vi "首页.vi"() -> ()   [LabVIEW 2016]
uses:
  <vilib>/Utility/miscctls.llb/LVPointTypeDef.ctl
  <vilib>/Utility/sysdir.llb/System Directory Type.ctl
  <vilib>/addons/database/_DB Variant To Data/Database Variant To Data.xnode
panel:
  out "显示":T1
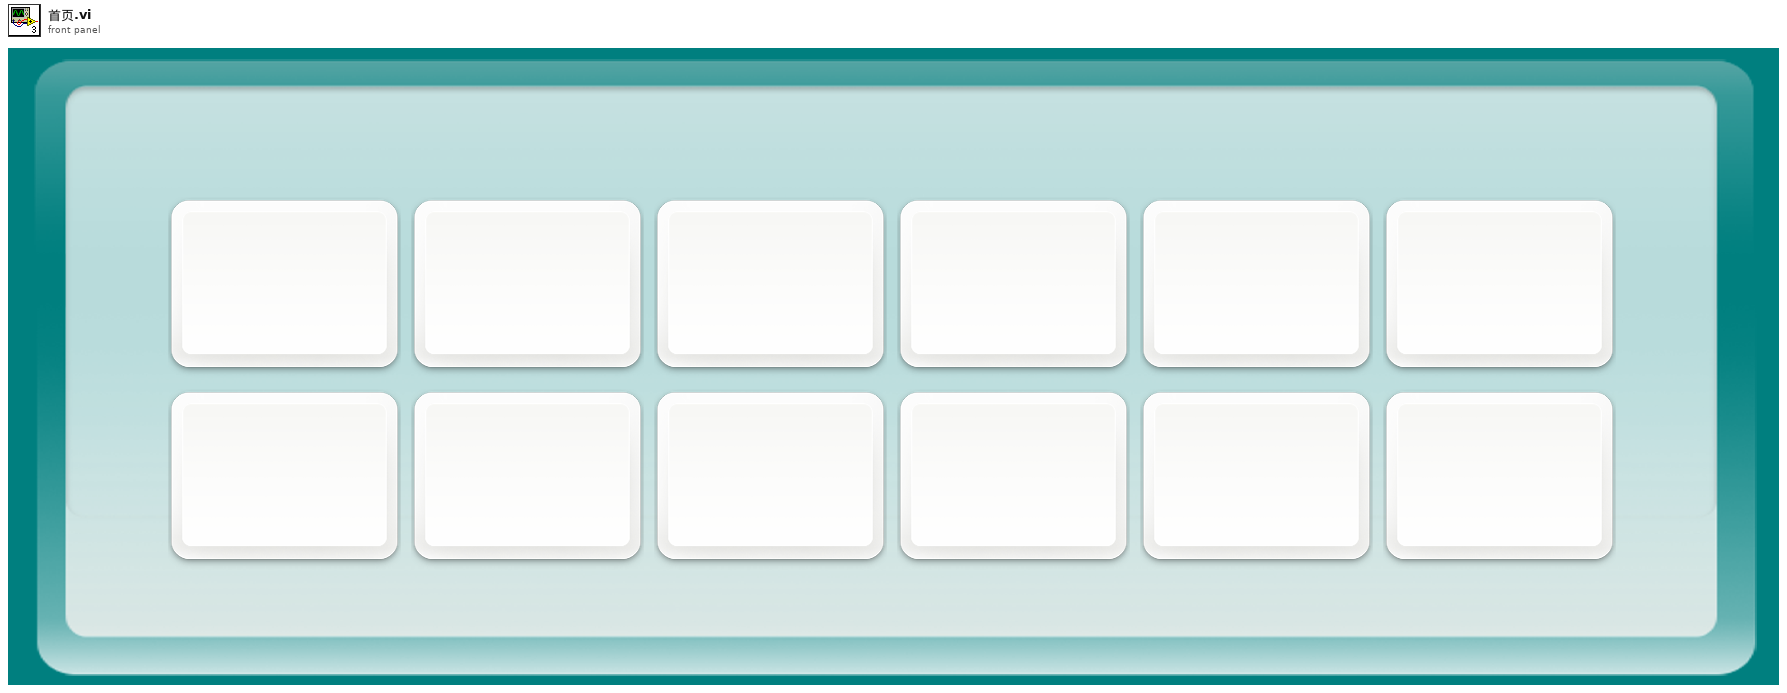
[diagram p1: front panel]
types:
  T1 = typedef "多数值显示.ctl" = cluster{"显示":T2, "显示 2":T2, "显示 3":T2, "显示 4":T2, "显示 5":T2, "显示 6":T2, "显示 12":T2, "显示 11":T2, "显示 10":T2, "显示 9":T2, "显示 8":T2, "显示 7":T2}
  T2 = typedef "数值显示.ctl" = cluster{"中文项目名称":string, "英文项目名称":string, "浓度":string, "单位":string}
  T3 = typedef "LVPointTypeDef.ctl" = cluster{"Horizontal":i16, "Vertical":i16}
  T4 = cluster{"显示参数中文名":string, "显示参数英文名":string, "显示浓度":string, "显示单位":string}[]
  T5 = cluster{"显示参数中文名":string, "显示参数英文名":string, "显示浓度":string, "显示单位":string}
  T6 = typedef "System Directory Type.ctl" = i32
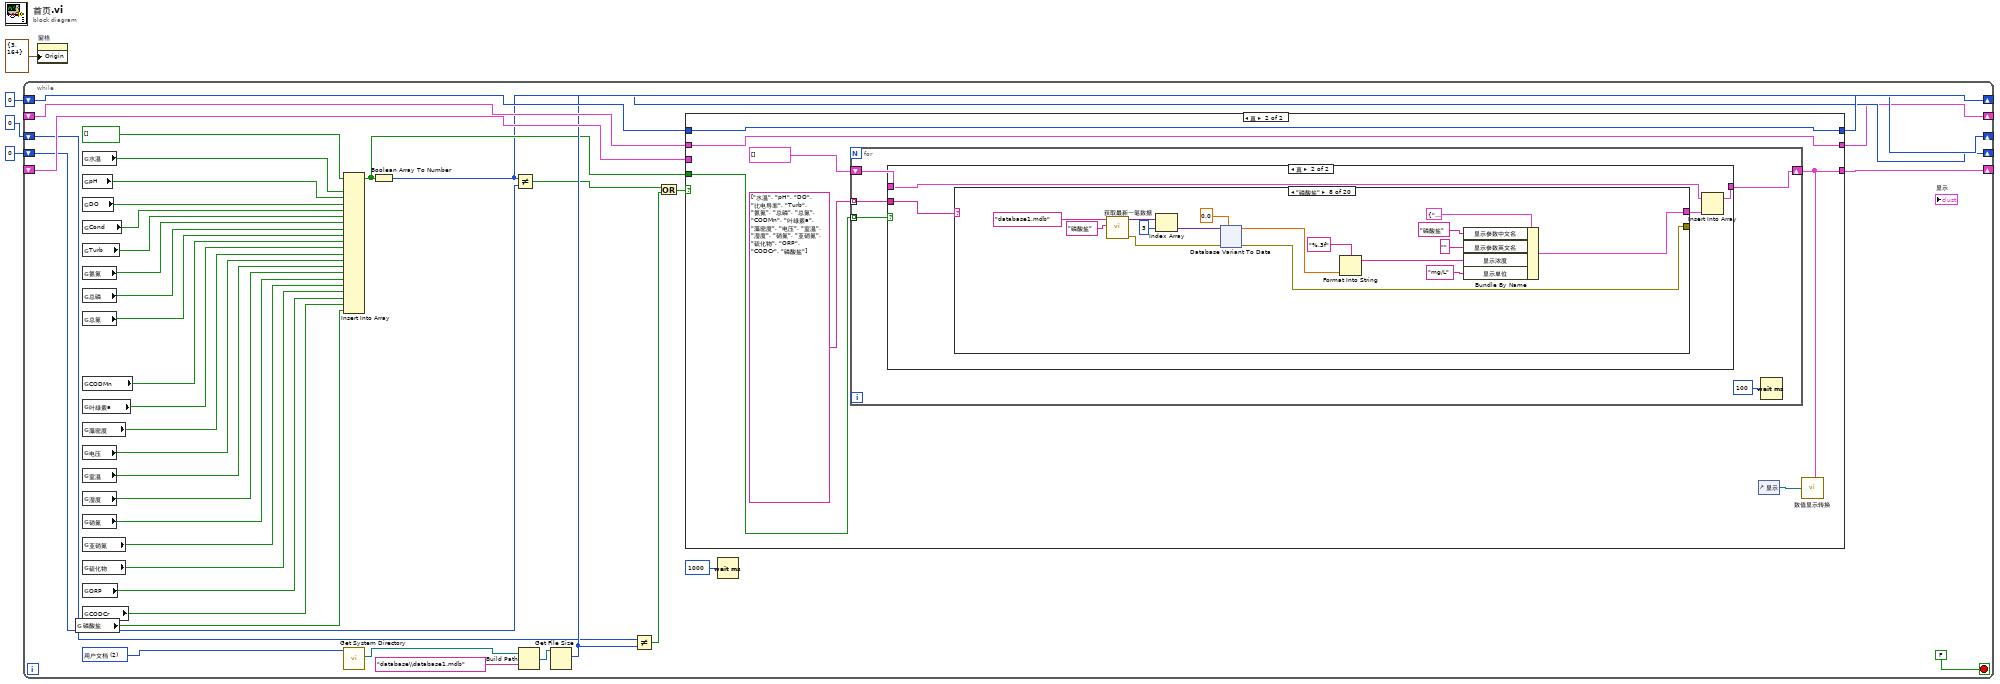
[diagram p0: block diagram]
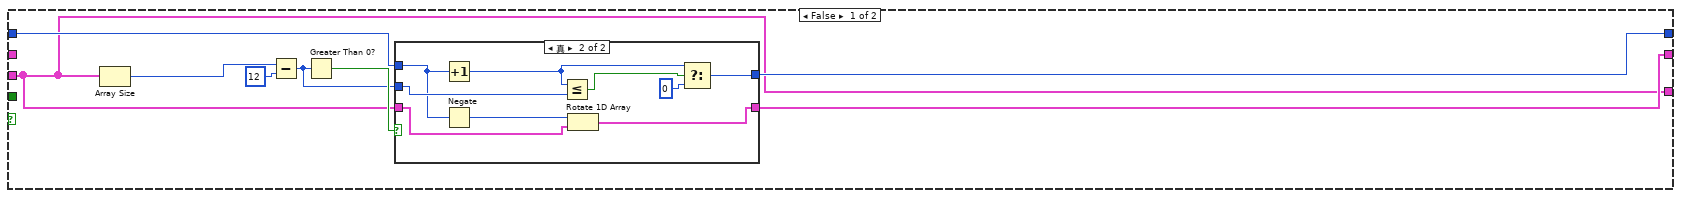
[diagram p2: hidden frame]
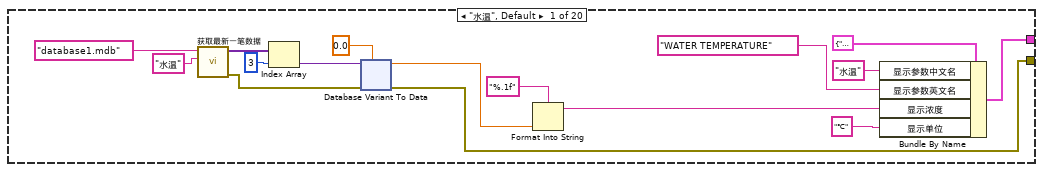
[diagram p5: hidden frame]
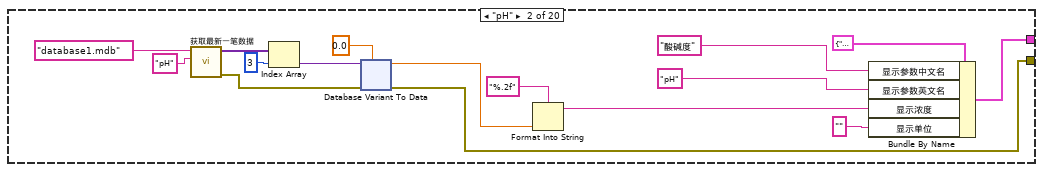
[diagram p6: hidden frame]
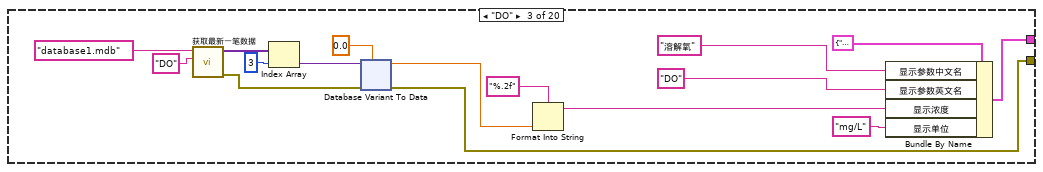
[diagram p7: hidden frame]
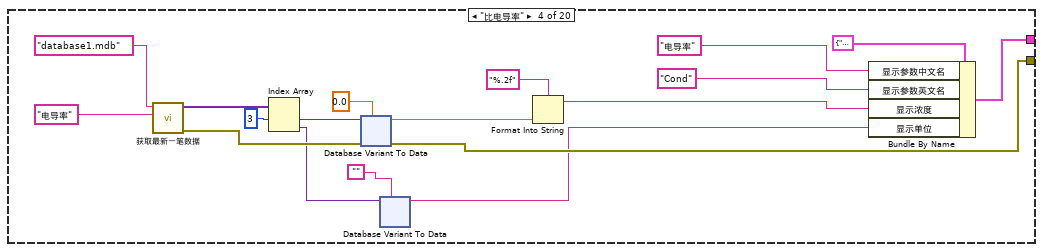
[diagram p8: hidden frame]
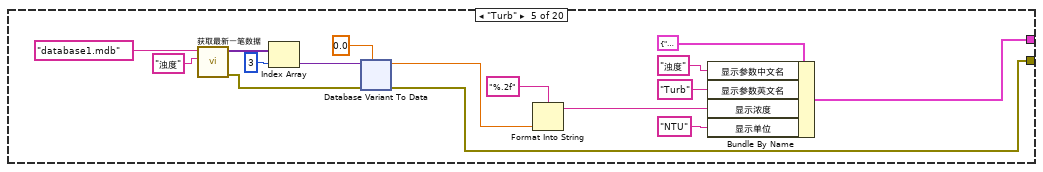
[diagram p9: hidden frame]
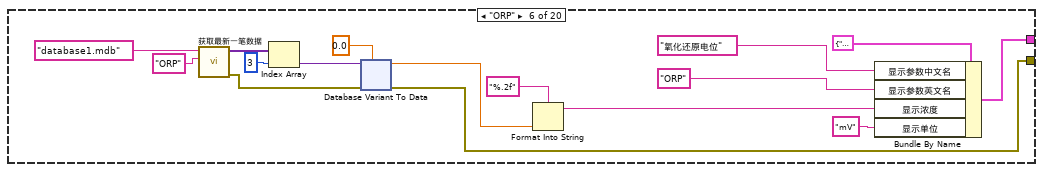
[diagram p10: hidden frame]
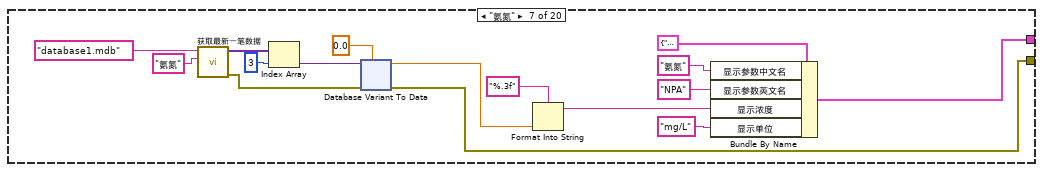
[diagram p11: hidden frame]
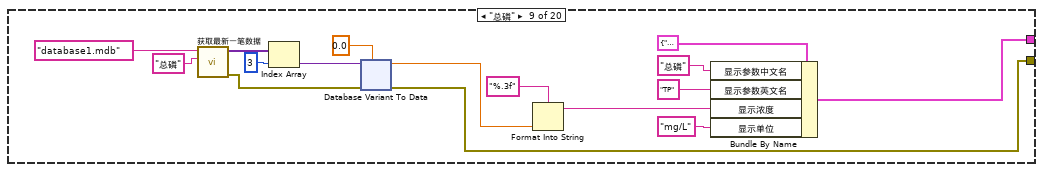
[diagram p12: hidden frame]
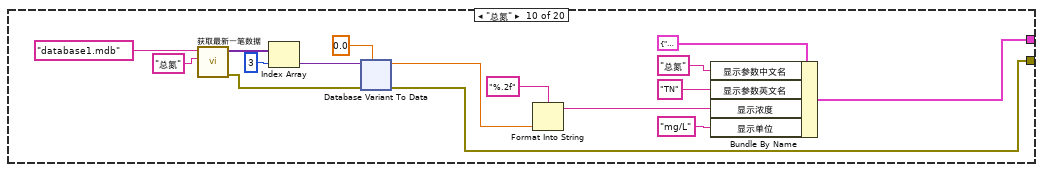
[diagram p13: hidden frame]
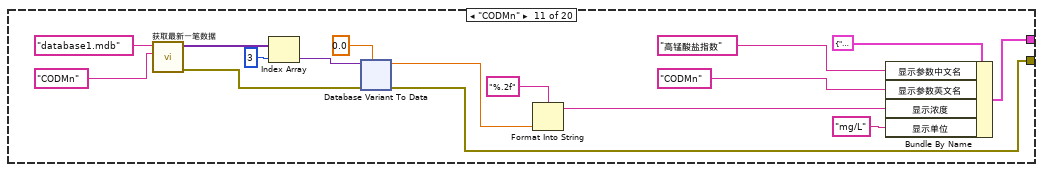
[diagram p14: hidden frame]
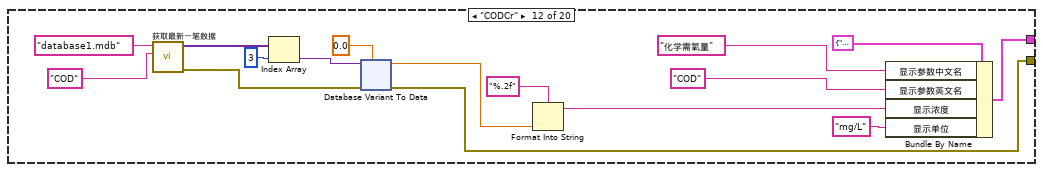
[diagram p15: hidden frame]
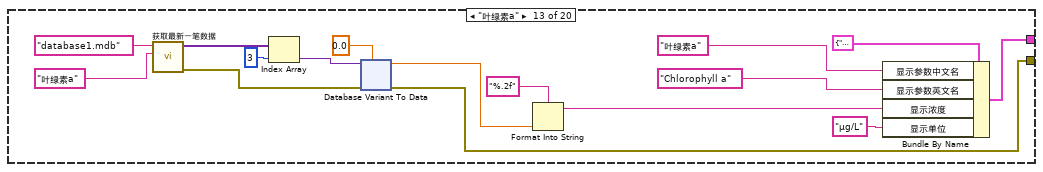
[diagram p16: hidden frame]
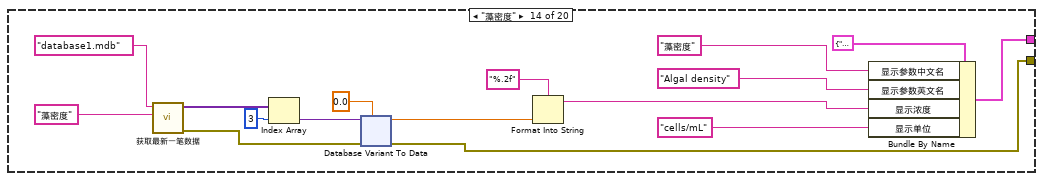
[diagram p17: hidden frame]
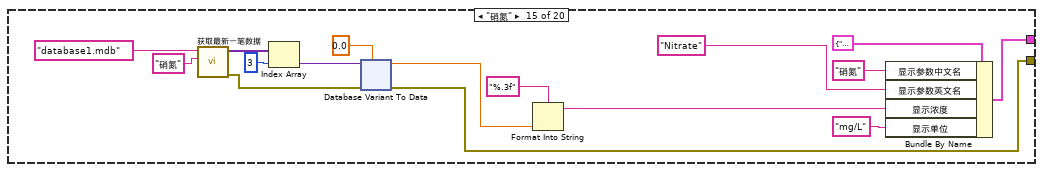
[diagram p18: hidden frame]
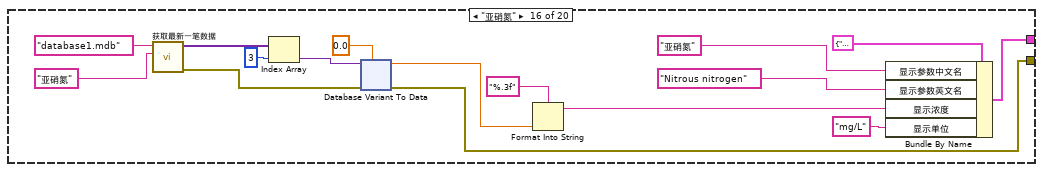
[diagram p19: hidden frame]
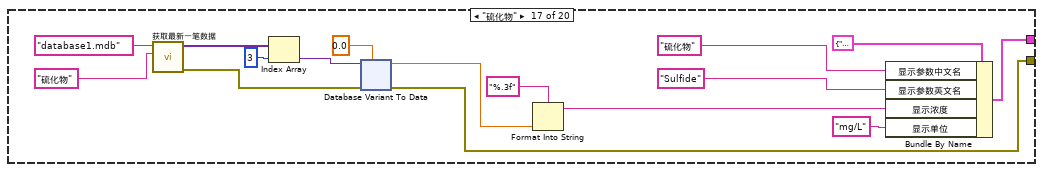
[diagram p20: hidden frame]
diagram:
  n1 = while {
    shift-right: [w43] -> _
    shift-left: _ -> [w42]
    shift-right: [w41] -> _
    shift-left: 0 -> [w44]
    shift-right: [w6] -> _
    shift-left: _ -> [w40]
    shift-right: [w35] -> _
    shift-left: i64 0 ("size (in bytes)") -> [w34]
    shift-right: [w13] -> _
    shift-left: u32 0 -> [w12]
    stop <- FALSE stop-if-true
    w39 = T6 2 items=["用户目录"=0, "用户桌面"=1, "用户文档"=2, "用户应用程序数据"=3, "用户设置"=4, "用户临时目录"=5, "公共文档"=6, "公共应用程序数据"=7, "公共设置"=8, "公共缓存"=13, "系统核心库"=9, "系统安装库"=10, "应用程序文件"=11, "启动盘根目录"=12] ("system directory type")
    n2 = global read "首页设置全局变量.vi" "磷酸盐"() -> (w5:bool)
    n3 = global read "首页设置全局变量.vi" "水温"() -> (w27:bool)
    n4 = global read "首页设置全局变量.vi" "pH"() -> (w26:bool)
    n5 = global read "首页设置全局变量.vi" "DO"() -> (w25:bool)
    n6 = global read "首页设置全局变量.vi" "Cond"() -> (w24:bool)
    n7 = global read "首页设置全局变量.vi" "Turb"() -> (w23:bool)
    n8 = global read "首页设置全局变量.vi" "氨氮"() -> (w22:bool)
    n9 = global read "首页设置全局变量.vi" "总磷"() -> (w21:bool)
    n10 = global read "首页设置全局变量.vi" "总氮"() -> (w20:bool)
    n11 = global read "首页设置全局变量.vi" "CODMn"() -> (w19:bool)
    n12 = global read "首页设置全局变量.vi" "叶绿素a"() -> (w18:bool)
    n13 = global read "首页设置全局变量.vi" "藻密度"() -> (w17:bool)
    n14 = global read "首页设置全局变量.vi" "电压"() -> (w16:bool)
    n15 = global read "首页设置全局变量.vi" "室温"() -> (w15:bool)
    n16 = global read "首页设置全局变量.vi" "湿度"() -> (w29:bool)
    n17 = global read "首页设置全局变量.vi" "硝氮"() -> (w30:bool)
    n18 = global read "首页设置全局变量.vi" "亚硝氮"() -> (w31:bool)
    n19 = global read "首页设置全局变量.vi" "硫化物"() -> (w32:bool)
    n20 = global read "首页设置全局变量.vi" "ORP"() -> (w33:bool)
    n21 = global read "首页设置全局变量.vi" "CODCr"() -> (w7:bool)
    n22 = Insert Into Array(array=bool[] [], new element #1=w27, new element #2=w26, new element #3=w25, new element #4=w24, new element #5=w23, new element #6=w22, new element #7=w21, new element #8=w20, new element #9=w19, new element #10=w18, new element #11=w17, new element #12=w16, new element #13=w15, new element #14=w29, new element #15=w30, new element #16=w31, new element #17=w32, new element #18=w33, new element #19=w7, new element #20=w5) -> (w14:bool[])  [unwired: 1 in]
    n23 = call <vilib>:"Get System Directory.vi"("system directory type"=w39) -> ("system directory"=w38:path)  [unwired: 10 in]
    n24 = Boolean Array To Number(Boolean array=w14) -> (number=w13:u32)
    n25 = Not Equal?(x=w13, y=w12) -> (x != y?=w11:bool)
    n26 = Build Path(base path=w38, name or relative path="database\\database1.mdb" ("名称或相对路径")) -> (appended path=w36:path)
    n27 = Get File Size(file=w36) -> (size (in bytes)=w35:i64)  [unwired: 1 in, 2 out]
    n28 = Not Equal?(x=w34, y=w35) -> (x != y?=w10:bool)
    n29 = Or(x=w11, y=w10) -> (x .or. y?=w9:bool)
    n30 = case shown="真" w9 {
      tunnel: w44 -> [w53 w68]
      tunnel: [w46 w64] -> w43
      tunnel: w42 -> [w46 _]
      tunnel: [w52 w68] -> w41
      tunnel: [w47 w67] -> w6
      tunnel: w40 -> [_ w67]
      tunnel: w14 -> [_ w66]
      frame False {
        n31 = Array Size(array=w46) -> (size(s)=w51:i32)
        n32 = Subtract(x=w51, y=12) -> (x-y=w48:i32)
        n33 = Greater Than 0?(x=w48) -> (x > 0?=w49:bool)
        n34 = case shown="真" w49 {
          tunnel: w46 -> [w54 w63]
          tunnel: w53 -> [_ w56]
          tunnel: [w54 w62] -> w47
          tunnel: [_ w57] -> w52
          tunnel: w48 -> [_ w60]
          frame False {
          }
          frame True {
            n35 = Increment(x=w56) -> (x+1=w61:i32)
            n36 = Negate(x=w56) -> (-x=w55:i32)
            n37 = Less Or Equal?(x=w61, y=w60) -> (x <= y?=w59:bool)
            n38 = Rotate 1D Array(1:w63, 2:w55) -> (0:w62:T4)
            n39 = Select(t=w61, s=w59, f=0) -> (s? t:f=w57:i32)
          }
        }
      }
      frame True {
        n40 = for {
          tunnel: w66 -> [w75] mode=indexing
          tunnel: string[] ["水温", "pH", "DO", "比电导率", "Turb", "氨氮", "总磷", "总氮", "CODMn", "叶绿素a", "藻密度", "电压", "室温", "湿度", "硝氮", "亚硝氮", "硫化物", "ORP", "CODCr", "磷酸盐"] -> [w74] mode=indexing
          shift-right: [w72] -> w64
          shift-left: T4 [] -> [w73]
          n41 = case shown="真" w75 {
            tunnel: w74 -> [_ w80]
            tunnel: w73 -> [w76 w79]
            tunnel: [w76 w78] -> w72
            frame False {
            }
            frame True {
              n42 = case shown="\"磷酸盐\"" w80 {
                tunnel: [w90 w140 w188 w239 w318 w366 w414 w462 w510 w558 w606 w654 w702 w750 w798 w846 w894 w934 w942 w950] -> w77
                tunnel: [w89 w137 w185 w235 w314 w362 w403 w451 w499 w547 w595 w643 w698 w739 w787 w835 w883 _ _ _] -> _
                frame "水温", Default {
                  n43 = call "获取最新一笔数据.vi"("table"="水温", "database"="database1.mdb" ("名称或相对路径")) -> ("error out"=w81:errorcluster, "子数组"=w86:variant[])  [unwired: 8 in]
                  n44 = Index Array(array=w86, index=3 ("索引")) -> (element=w84:variant)
                  n45 = xnode "Database Variant To Data"("database variant"=w84, "error in (no error)"=w81, "type"=0.0) -> ("data"=w88:dbl, "error out"=w89:errorcluster)
                  n46 = Format Into String(format string="%.1f" ("格式字符串"), w88) -> (resulting string=w91:string)  [unwired: 2 in, 1 out]
                  n47 = Bundle By Name(cluster=T5 {"显示参数中文名"="", "显示参数英文名"="", "显示浓度"="", "显示单位"=""} ("元素"), "显示参数中文名"="水温", "显示参数英文名"="WATER TEMPERATURE", "显示浓度"=w91, "显示单位"="℃") -> (w90:T5)
                }
                frame "pH" {
                  n48 = call "获取最新一笔数据.vi"("table"="pH", "database"="database1.mdb" ("名称或相对路径")) -> ("error out"=w129:errorcluster, "子数组"=w134:variant[])  [unwired: 8 in]
                  n49 = Index Array(array=w134, index=3 ("索引")) -> (element=w132:variant)
                  n50 = xnode "Database Variant To Data"("database variant"=w132, "error in (no error)"=w129, "type"=0.0) -> ("data"=w136:dbl, "error out"=w137:errorcluster)
                  n51 = Format Into String(format string="%.2f" ("格式字符串"), w136) -> (resulting string=w138:string)  [unwired: 2 in, 1 out]
                  n52 = Bundle By Name(cluster=T5 {"显示参数中文名"="", "显示参数英文名"="", "显示浓度"="", "显示单位"=""} ("元素"), "显示参数中文名"="酸碱度", "显示参数英文名"="pH", "显示浓度"=w138, "显示单位"="") -> (w140:T5)
                }
                frame "DO" {
                  n53 = call "获取最新一笔数据.vi"("table"="DO", "database"="database1.mdb" ("名称或相对路径")) -> ("error out"=w177:errorcluster, "子数组"=w182:variant[])  [unwired: 8 in]
                  n54 = Index Array(array=w182, index=3 ("索引")) -> (element=w180:variant)
                  n55 = xnode "Database Variant To Data"("database variant"=w180, "error in (no error)"=w177, "type"=0.0) -> ("data"=w184:dbl, "error out"=w185:errorcluster)
                  n56 = Format Into String(format string="%.2f" ("格式字符串"), w184) -> (resulting string=w186:string)  [unwired: 2 in, 1 out]
                  n57 = Bundle By Name(cluster=T5 {"显示参数中文名"="", "显示参数英文名"="", "显示浓度"="", "显示单位"=""} ("元素"), "显示参数中文名"="溶解氧", "显示参数英文名"="DO", "显示浓度"=w186, "显示单位"="mg/L") -> (w188:T5)
                }
                frame "比电导率" {
                  n58 = call "获取最新一笔数据.vi"("table"="电导率", "database"="database1.mdb" ("名称或相对路径")) -> ("error out"=w228:errorcluster, "子数组"=w233:variant[])  [unwired: 8 in]
                  n59 = Index Array(array=w233, index #1=3 ("索引")) -> (element #1=w231:variant, element #2=w227:variant)  [unwired: 1 in]
                  n60 = xnode "Database Variant To Data"("database variant"=w231, "error in (no error)"=w228, "type"=0.0) -> ("data"=w236:dbl, "error out"=w235:errorcluster)
                  n61 = xnode "Database Variant To Data"("database variant"=w227, "type"="") -> ("data"=w225:string)  [unwired: 1 in, 1 out]
                  n62 = Format Into String(format string="%.2f" ("格式字符串"), w236) -> (resulting string=w237:string)  [unwired: 2 in, 1 out]
                  n63 = Bundle By Name(cluster=T5 {"显示参数中文名"="", "显示参数英文名"="", "显示浓度"="", "显示单位"=""} ("元素"), "显示参数中文名"="电导率", "显示参数英文名"="Cond", "显示浓度"=w237, "显示单位"=w225) -> (w239:T5)
                }
                frame "Turb" {
                  n64 = call "获取最新一笔数据.vi"("table"="浊度", "database"="database1.mdb" ("名称或相对路径")) -> ("error out"=w307:errorcluster, "子数组"=w312:variant[])  [unwired: 8 in]
                  n65 = Index Array(array=w312, index=3 ("索引")) -> (element=w310:variant)
                  n66 = xnode "Database Variant To Data"("database variant"=w310, "error in (no error)"=w307, "type"=0.0) -> ("data"=w315:dbl, "error out"=w314:errorcluster)
                  n67 = Format Into String(format string="%.2f" ("格式字符串"), w315) -> (resulting string=w316:string)  [unwired: 2 in, 1 out]
                  n68 = Bundle By Name(cluster=T5 {"显示参数中文名"="", "显示参数英文名"="", "显示浓度"="", "显示单位"=""} ("元素"), "显示参数中文名"="浊度", "显示参数英文名"="Turb", "显示浓度"=w316, "显示单位"="NTU") -> (w318:T5)
                }
                frame "ORP" {
                  n69 = call "获取最新一笔数据.vi"("table"="ORP", "database"="database1.mdb" ("名称或相对路径")) -> ("error out"=w355:errorcluster, "子数组"=w360:variant[])  [unwired: 8 in]
                  n70 = Index Array(array=w360, index=3 ("索引")) -> (element=w358:variant)
                  n71 = xnode "Database Variant To Data"("database variant"=w358, "error in (no error)"=w355, "type"=0.0) -> ("data"=w363:dbl, "error out"=w362:errorcluster)
                  n72 = Format Into String(format string="%.2f" ("格式字符串"), w363) -> (resulting string=w364:string)  [unwired: 2 in, 1 out]
                  n73 = Bundle By Name(cluster=T5 {"显示参数中文名"="", "显示参数英文名"="", "显示浓度"="", "显示单位"=""} ("元素"), "显示参数中文名"="氧化还原电位", "显示参数英文名"="ORP", "显示浓度"=w364, "显示单位"="mV") -> (w366:T5)
                }
                frame "氨氮" {
                  n74 = call "获取最新一笔数据.vi"("table"="氨氮", "database"="database1.mdb" ("名称或相对路径")) -> ("error out"=w404:errorcluster, "子数组"=w410:variant[])  [unwired: 8 in]
                  n75 = Index Array(array=w410, index=3 ("索引")) -> (element=w408:variant)
                  n76 = xnode "Database Variant To Data"("database variant"=w408, "error in (no error)"=w404, "type"=0.0) -> ("data"=w405:dbl, "error out"=w403:errorcluster)
                  n77 = Format Into String(format string="%.3f" ("格式字符串"), w405) -> (resulting string=w412:string)  [unwired: 2 in, 1 out]
                  n78 = Bundle By Name(cluster=T5 {"显示参数中文名"="", "显示参数英文名"="", "显示浓度"="", "显示单位"=""} ("元素"), "显示参数中文名"="氨氮", "显示参数英文名"="NPA", "显示浓度"=w412, "显示单位"="mg/L") -> (w414:T5)
                }
                frame "磷酸盐" {
                  n79 = call "获取最新一笔数据.vi"("table"="磷酸盐", "database"="database1.mdb" ("名称或相对路径")) -> ("error out"=w452:errorcluster, "子数组"=w458:variant[])  [unwired: 8 in]
                  n80 = Index Array(array=w458, index=3 ("索引")) -> (element=w456:variant)
                  n81 = xnode "Database Variant To Data"("database variant"=w456, "error in (no error)"=w452, "type"=0.0) -> ("data"=w453:dbl, "error out"=w451:errorcluster)
                  n82 = Format Into String(format string="%.3f" ("格式字符串"), w453) -> (resulting string=w460:string)  [unwired: 2 in, 1 out]
                  n83 = Bundle By Name(cluster=T5 {"显示参数中文名"="", "显示参数英文名"="", "显示浓度"="", "显示单位"=""} ("元素"), "显示参数中文名"="磷酸盐", "显示参数英文名"="", "显示浓度"=w460, "显示单位"="mg/L") -> (w462:T5)
                }
                frame "总磷" {
                  n84 = call "获取最新一笔数据.vi"("table"="总磷", "database"="database1.mdb" ("名称或相对路径")) -> ("error out"=w500:errorcluster, "子数组"=w506:variant[])  [unwired: 8 in]
                  n85 = Index Array(array=w506, index=3 ("索引")) -> (element=w504:variant)
                  n86 = xnode "Database Variant To Data"("database variant"=w504, "error in (no error)"=w500, "type"=0.0) -> ("data"=w501:dbl, "error out"=w499:errorcluster)
                  n87 = Format Into String(format string="%.3f" ("格式字符串"), w501) -> (resulting string=w508:string)  [unwired: 2 in, 1 out]
                  n88 = Bundle By Name(cluster=T5 {"显示参数中文名"="", "显示参数英文名"="", "显示浓度"="", "显示单位"=""} ("元素"), "显示参数中文名"="总磷", "显示参数英文名"="TP", "显示浓度"=w508, "显示单位"="mg/L") -> (w510:T5)
                }
                frame "总氮" {
                  n89 = call "获取最新一笔数据.vi"("table"="总氮", "database"="database1.mdb" ("名称或相对路径")) -> ("error out"=w548:errorcluster, "子数组"=w554:variant[])  [unwired: 8 in]
                  n90 = Index Array(array=w554, index=3 ("索引")) -> (element=w552:variant)
                  n91 = xnode "Database Variant To Data"("database variant"=w552, "error in (no error)"=w548, "type"=0.0) -> ("data"=w549:dbl, "error out"=w547:errorcluster)
                  n92 = Format Into String(format string="%.2f" ("格式字符串"), w549) -> (resulting string=w556:string)  [unwired: 2 in, 1 out]
                  n93 = Bundle By Name(cluster=T5 {"显示参数中文名"="", "显示参数英文名"="", "显示浓度"="", "显示单位"=""} ("元素"), "显示参数中文名"="总氮", "显示参数英文名"="TN", "显示浓度"=w556, "显示单位"="mg/L") -> (w558:T5)
                }
                frame "CODMn" {
                  n94 = call "获取最新一笔数据.vi"("table"="CODMn", "database"="database1.mdb" ("名称或相对路径")) -> ("error out"=w596:errorcluster, "子数组"=w602:variant[])  [unwired: 8 in]
                  n95 = Index Array(array=w602, index=3 ("索引")) -> (element=w600:variant)
                  n96 = xnode "Database Variant To Data"("database variant"=w600, "error in (no error)"=w596, "type"=0.0) -> ("data"=w597:dbl, "error out"=w595:errorcluster)
                  n97 = Format Into String(format string="%.2f" ("格式字符串"), w597) -> (resulting string=w604:string)  [unwired: 2 in, 1 out]
                  n98 = Bundle By Name(cluster=T5 {"显示参数中文名"="", "显示参数英文名"="", "显示浓度"="", "显示单位"=""} ("元素"), "显示参数中文名"="高锰酸盐指数", "显示参数英文名"="CODMn", "显示浓度"=w604, "显示单位"="mg/L") -> (w606:T5)
                }
                frame "CODCr" {
                  n99 = call "获取最新一笔数据.vi"("table"="COD", "database"="database1.mdb" ("名称或相对路径")) -> ("error out"=w644:errorcluster, "子数组"=w650:variant[])  [unwired: 8 in]
                  n100 = Index Array(array=w650, index=3 ("索引")) -> (element=w648:variant)
                  n101 = xnode "Database Variant To Data"("database variant"=w648, "error in (no error)"=w644, "type"=0.0) -> ("data"=w645:dbl, "error out"=w643:errorcluster)
                  n102 = Format Into String(format string="%.2f" ("格式字符串"), w645) -> (resulting string=w652:string)  [unwired: 2 in, 1 out]
                  n103 = Bundle By Name(cluster=T5 {"显示参数中文名"="", "显示参数英文名"="", "显示浓度"="", "显示单位"=""} ("元素"), "显示参数中文名"="化学需氧量", "显示参数英文名"="COD", "显示浓度"=w652, "显示单位"="mg/L") -> (w654:T5)
                }
                frame "叶绿素a" {
                  n104 = call "获取最新一笔数据.vi"("table"="叶绿素a", "database"="database1.mdb" ("名称或相对路径")) -> ("error out"=w691:errorcluster, "子数组"=w696:variant[])  [unwired: 8 in]
                  n105 = Index Array(array=w696, index=3 ("索引")) -> (element=w694:variant)
                  n106 = xnode "Database Variant To Data"("database variant"=w694, "error in (no error)"=w691, "type"=0.0) -> ("data"=w699:dbl, "error out"=w698:errorcluster)
                  n107 = Format Into String(format string="%.2f" ("格式字符串"), w699) -> (resulting string=w700:string)  [unwired: 2 in, 1 out]
                  n108 = Bundle By Name(cluster=T5 {"显示参数中文名"="", "显示参数英文名"="", "显示浓度"="", "显示单位"=""} ("元素"), "显示参数中文名"="叶绿素a", "显示参数英文名"="Chlorophyll a", "显示浓度"=w700, "显示单位"="μg/L") -> (w702:T5)
                }
                frame "藻密度" {
                  n109 = call "获取最新一笔数据.vi"("table"="藻密度", "database"="database1.mdb" ("名称或相对路径")) -> ("error out"=w740:errorcluster, "子数组"=w746:variant[])  [unwired: 8 in]
                  n110 = Index Array(array=w746, index=3 ("索引")) -> (element=w744:variant)
                  n111 = xnode "Database Variant To Data"("database variant"=w744, "error in (no error)"=w740, "type"=0.0) -> ("data"=w741:dbl, "error out"=w739:errorcluster)
                  n112 = Format Into String(format string="%.2f" ("格式字符串"), w741) -> (resulting string=w748:string)  [unwired: 2 in, 1 out]
                  n113 = Bundle By Name(cluster=T5 {"显示参数中文名"="", "显示参数英文名"="", "显示浓度"="", "显示单位"=""} ("元素"), "显示参数中文名"="藻密度", "显示参数英文名"="Algal density", "显示浓度"=w748, "显示单位"="cells/mL") -> (w750:T5)
                }
                frame "硝氮" {
                  n114 = call "获取最新一笔数据.vi"("table"="硝氮", "database"="database1.mdb" ("名称或相对路径")) -> ("error out"=w788:errorcluster, "子数组"=w794:variant[])  [unwired: 8 in]
                  n115 = Index Array(array=w794, index=3 ("索引")) -> (element=w792:variant)
                  n116 = xnode "Database Variant To Data"("database variant"=w792, "error in (no error)"=w788, "type"=0.0) -> ("data"=w789:dbl, "error out"=w787:errorcluster)
                  n117 = Format Into String(format string="%.3f" ("格式字符串"), w789) -> (resulting string=w796:string)  [unwired: 2 in, 1 out]
                  n118 = Bundle By Name(cluster=T5 {"显示参数中文名"="", "显示参数英文名"="", "显示浓度"="", "显示单位"=""} ("元素"), "显示参数中文名"="硝氮", "显示参数英文名"="Nitrate", "显示浓度"=w796, "显示单位"="mg/L") -> (w798:T5)
                }
                frame "亚硝氮" {
                  n119 = call "获取最新一笔数据.vi"("table"="亚硝氮", "database"="database1.mdb" ("名称或相对路径")) -> ("error out"=w836:errorcluster, "子数组"=w842:variant[])  [unwired: 8 in]
                  n120 = Index Array(array=w842, index=3 ("索引")) -> (element=w840:variant)
                  n121 = xnode "Database Variant To Data"("database variant"=w840, "error in (no error)"=w836, "type"=0.0) -> ("data"=w837:dbl, "error out"=w835:errorcluster)
                  n122 = Format Into String(format string="%.3f" ("格式字符串"), w837) -> (resulting string=w844:string)  [unwired: 2 in, 1 out]
                  n123 = Bundle By Name(cluster=T5 {"显示参数中文名"="", "显示参数英文名"="", "显示浓度"="", "显示单位"=""} ("元素"), "显示参数中文名"="亚硝氮", "显示参数英文名"="Nitrous nitrogen", "显示浓度"=w844, "显示单位"="mg/L") -> (w846:T5)
                }
                frame "硫化物" {
                  n124 = call "获取最新一笔数据.vi"("table"="硫化物", "database"="database1.mdb" ("名称或相对路径")) -> ("error out"=w884:errorcluster, "子数组"=w890:variant[])  [unwired: 8 in]
                  n125 = Index Array(array=w890, index=3 ("索引")) -> (element=w888:variant)
                  n126 = xnode "Database Variant To Data"("database variant"=w888, "error in (no error)"=w884, "type"=0.0) -> ("data"=w885:dbl, "error out"=w883:errorcluster)
                  n127 = Format Into String(format string="%.3f" ("格式字符串"), w885) -> (resulting string=w892:string)  [unwired: 2 in, 1 out]
                  n128 = Bundle By Name(cluster=T5 {"显示参数中文名"="", "显示参数英文名"="", "显示浓度"="", "显示单位"=""} ("元素"), "显示参数中文名"="硫化物", "显示参数英文名"="Sulfide", "显示浓度"=w892, "显示单位"="mg/L") -> (w894:T5)
                }
                frame "电压" {
                  n129 = Format Into String(format string="%.2f" ("格式字符串"), 0.0 ("输入 1")) -> (resulting string=w932:string)  [unwired: 2 in, 1 out]
                  n130 = Bundle By Name(cluster=T5 {"显示参数中文名"="", "显示参数英文名"="", "显示浓度"="", "显示单位"=""} ("元素"), "显示参数中文名"="电压", "显示参数英文名"="Voltage", "显示浓度"=w932, "显示单位"="V") -> (w934:T5)
                }
                frame "室温" {
                  n131 = Format Into String(format string="%.2f" ("格式字符串"), 0.0 ("输入 1")) -> (resulting string=w940:string)  [unwired: 2 in, 1 out]
                  n132 = Bundle By Name(cluster=T5 {"显示参数中文名"="", "显示参数英文名"="", "显示浓度"="", "显示单位"=""} ("元素"), "显示参数中文名"="室温", "显示参数英文名"="Room temperature", "显示浓度"=w940, "显示单位"="℃") -> (w942:T5)
                }
                frame "湿度" {
                  n133 = Format Into String(format string="%.2f" ("格式字符串"), 0.0 ("输入 1")) -> (resulting string=w948:string)  [unwired: 2 in, 1 out]
                  n134 = Bundle By Name(cluster=T5 {"显示参数中文名"="", "显示参数英文名"="", "显示浓度"="", "显示单位"=""} ("元素"), "显示参数中文名"="湿度", "显示参数英文名"="humidity", "显示浓度"=w948, "显示单位"="%RH") -> (w950:T5)
                }
              }
              n135 = Insert Into Array(array=w79, new element=w77) -> (w78:T4)  [unwired: 1 in]
            }
          }
          n136 = Wait (ms)(milliseconds to wait=u32 100 ("等待时间（毫秒）")) -> ()  [unwired: 1 out]
        }
        n137 = control-ref of="显示"() -> (w65:refnum<vi>)
        n138 = call "数值显示转换.vi"("显示"=w65, "数组"=w64) -> ()  [unwired: 10 in]
      }
    }
    n139 = Wait (ms)(milliseconds to wait=u32 1000 ("等待时间（毫秒）")) -> ()  [unwired: 1 out]
  }
  n140 = property on="窗格" class="Pane"("Origin"=T3 {"Horizontal"=3, "Vertical"=164} ("原点")) -> ()  [unwired: 2 in, 2 out]
